vi "PicoScope4000aExampleBlock_PicoConnect.vi"() -> ()   [LabVIEW 2010]
doc: "This example demonstrates how to use the PicoScope Labview library to collect data using block mode with PicoConnect probe infomation."
uses:
  shared/PicoBuffers.ctl
  PicoScope4000aLib/PicoScope4000aAnalogChannelSettings_PicoConnect.ctl
  shared/Buffer and Transfer Settings.ctl
  shared/Acquisition Settings.ctl
panel:
  in  "Range":u32(ring)=4000 items=["10mV"=0, "20mV"=1, "50mV"=2, "100mV"=3, "200mV"=4, "500mV"=5, "1V"=6, "2V"=7, "5V"=8, "10V"=9, "20V"=10, "50V"=11, "100V"=12, "200V"=13, "1KV_2_5V"=6003, "1KV_5V"=6004, "1KV_12_5V"=6005, "1KV_25V"=6006, "1KV_50V"=6007, "1KV_125V"=6008, "1KV_250V"=6009, "1KV_500V"=6010, "1KV_1000V"=6011, "CURRENT_CLAMP_200A_2kA_1A"=4000, "CURRENT_CLAMP_200A_2kA_2A"=4001, "CURRENT_CLAMP_200A_2kA_5A"=4002, "CURRENT_CLAMP_200A_2kA_10A"=4003, "CURRENT_CLAMP_200A_2kA_20A"=4004, "CURRENT_CLAMP_200A_2kA_50A"=4005, "CURRENT_CLAMP_200A_2kA_100A"=4006, "CURRENT_CLAMP_200A_2kA_200A"=4007, "CURRENT_CLAMP_200A_2kA_500A"=4008, "CURRENT_CLAMP_200A_2kA_1000A"=4009, "CURRENT_CLAMP_200A_2kA_2000A"=4010, "CURRENT_CLAMP_40A_100mA"=5000, "CURRENT_CLAMP_40A_200mA"=5001, "CURRENT_CLAMP_40A_500mA"=5002, "CURRENT_CLAMP_40A_1A"=5003, "CURRENT_CLAMP_40A_2A"=5004, "CURRENT_CLAMP_40A_5A"=5005, "CURRENT_CLAMP_40A_10A"=5006, "CURRENT_CLAMP_40A_20A"=5007, "CURRENT_CLAMP_40A_40A"=5008, "CURRENT_CLAMP_2000ARMS_10A"=6500, "CURRENT_CLAMP_2000ARMS_20A"=6501, "CURRENT_CLAMP_2000ARMS_50A"=6502, "CURRENT_CLAMP_2000ARMS_100A"=6503, "CURRENT_CLAMP_2000ARMS_200A"=6504, "CURRENT_CLAMP_2000ARMS_500A"=6505, "CURRENT_CLAMP_2000ARMS_1000A"=6506, "CURRENT_CLAMP_2000ARMS_2000A"=6507, "CURRENT_CLAMP_2000ARMS_5000A"=6508, "x10_Probe_100mV"=32, "x10_Probe_200mV"=33, "x10_Probe_500mV"=34, "x10_Probe_1V"=35, "x10_Probe_2V"=36, "x10_Probe_5V"=37, "x10_Probe_10V"=38, "x10_Probe_20V"=39, "x10_Probe_50V"=40, "x10_Probe_100V"=41, "x10_Probe_200V"=42, "x10_Probe_500V"=43, "CURRENT_CLAMP_60A_2A"=10500, "CURRENT_CLAMP_60A_5A"=10501, "CURRENT_CLAMP_60A_10A"=10502, "CURRENT_CLAMP_60A_20A"=10503, "CURRENT_CLAMP_60A_50A"=10504, "CURRENT_CLAMP_60A_60A"=10505, "CURRENT_CLAMP_60A_V2_0_5A"=10600, "CURRENT_CLAMP_60A_V2_1A"=10601, "CURRENT_CLAMP_60A_V2_2A"=10602, "CURRENT_CLAMP_60A_V2_5A"=10603, "CURRENT_CLAMP_60A_V2_10A"=10604, "CURRENT_CLAMP_60A_V2_20A"=10605, "CURRENT_CLAMP_60A_V2_50A"=10606, "CURRENT_CLAMP_60A_V2_60A"=10607, "RESISTANCE_LEAD_NEG5_TO_20OHM"=7000, "RESISTANCE_LEAD_NEG50_TO_200OHM"=7001, "RESISTANCE_LEAD_NEG500_TO_2KOHM"=7002, "RESISTANCE_LEAD_NEG5K_TO_20KOHM"=7003, "RESISTANCE_LEAD_NEG50K_TO_LEAD_200KOHM"=7004, "RESISTANCE_LEAD_NEG500K_TO_LEAD_2MOHM"=7005, "RESISTANCE_LEAD_DIODE_TEST"=7006, "HT_NEG3_TO_5KV"=8950, "HT_NEG3_TO_10KV"=8951, "HT_NEG5_TO_20KV"=8952, "HT_NEG5_TO_50KV"=8953, "HT_NEG5_TO_100KV"=8954, "HT_NEG3_TO_5KV_INVERTED"=8955, "HT_NEG3_TO_10KV_INVERTED"=8956, "HT_NEG5_TO_20KV_INVERTED"=8957, "HT_NEG5_TO_50KV_INVERTED"=8958, "HT_NEG5_TO_100KV_INVERTED"=8959, "TEMPERATURE_NEG50_TO_150DEGC"=9000, "PRESSURE_SENSOR_-100k-150k_PASCALS"=9100, "PRESSURE_SENSOR_-100k_TO_400k_PASCALS"=9101, "PRESSURE_SENSOR_-200k_TO_800k_PASCALS"=9102, "PRESSURE_SENSOR_-400k_TO_1600k_PASCALS"=9103, "PRESSURE_SENSOR_-400k_TO_3400k_PASCALS"=9104, "PRESSURE_SENSOR_-150k_TO_1350k_PASCALS"=9105]
  in  "Trigger Settings":T1={"Trigger Enabled"=FALSE, "Trigger Source"=enum."Channel A", "Trigger Threshold (Volts/Probe units)"=0.0, "Trigger Direction"=2, "Trigger Delay (samples)"=0, "Auto Trigger Time (ms)"=1000} {"Trigger Direction" items=["Above", "Below", "Rising", "Falling", "Rising or Falling"]}
  out "Unit Info":T2
  out "minimumValue":sgl
  out "maximumValue":sgl
  out "Channel B":cluster{i32, dbl, "Data":dbl[]}[](graph)
  in  "Acquisition Settings":T3={"preTriggerSamples"=0, "postTriggerSamples"=5000000, "timebase"=5} {"postTriggerSamples" format="%_6p"; "preTriggerSamples" format="%_6p"}
  in  "Buffer and Transfer Settings":T4={"startIndex"=0, "Samples"=5000000, "Down Sample Ratio"=1, "Down-Sample Mode"=0} {"Down-Sample Mode" items=["RAW none"=2147483648, "None"=0, "Aggregate"=1, "Decimate"=2, "Average"=4]; "Down Sample Ratio" step=1; "Samples" format="%_6p"}
  out "Properties Panel":T5 {"Max Total Capture Time Available (sec)" format="%.3p"; "Sample Frequency" format="%.6p"; "Sample Rate" format="%.3p"; "Max Samples Available" format="%_6p"; "Total Capture Time (sec)" format="%.3p"}
  out "overflow":i16 format="%04b"
  out "Channel A":cluster{i32, dbl, "Data":dbl[]}(graph)
  in  "stop":bool
  out "ChB Probe":i32(ring) items=["CONNECT_PROBE_NONE"=0, "PROBE_D9_BNC"=4000, "PROBE_D9_2X_BNC"=4001, "PROBE_DIFFERENTIAL"=4002, "PROBE_CURRENT_CLAMP_200_2KA"=4003, "CONNECT_PROBE_CURRENT_CLAMP_40A"=4004, "CONNECT_PROBE_CAT3_HV_1KV"=4005, "CONNECT_PROBE_CURRENT_CLAMP_2000ARMS"=4006, "CONNECT_PROBE_INTELLIGENT"=-3, "CONNECT_PROBE_FAULT_PROBE"=-1, "CONNECT_PROBE_UNKNOWN_PROBE"=-2]
  in  "Channel A Settings":T6={"Enabled"=TRUE, "Coupling"=1, "Range"=0, "Analogue Offset"=0.0, "Bandwidth Limit"=0} {"Range" items=["10mV"=0, "20mV"=1, "50mV"=2, "100mV"=3, "200mV"=4, "500mV"=5, "1V"=6, "2V"=7, "5V"=8, "10V"=9, "20V"=10, "50V"=11, "100V"=12, "200V"=13, "1KV_2_5V"=6003, "1KV_5V"=6004, "1KV_12_5V"=6005, "1KV_25V"=6006, "1KV_50V"=6007, "1KV_125V"=6008, "1KV_250V"=6009, "1KV_500V"=6010, "1KV_1000V"=6011, "CURRENT_CLAMP_200A_2kA_1A"=4000, "CURRENT_CLAMP_200A_2kA_2A"=4001, "CURRENT_CLAMP_200A_2kA_5A"=4002, "CURRENT_CLAMP_200A_2kA_10A"=4003, "CURRENT_CLAMP_200A_2kA_20A"=4004, "CURRENT_CLAMP_200A_2kA_50A"=4005, "CURRENT_CLAMP_200A_2kA_100A"=4006, "CURRENT_CLAMP_200A_2kA_200A"=4007, "CURRENT_CLAMP_200A_2kA_500A"=4008, "CURRENT_CLAMP_200A_2kA_1000A"=4009, "CURRENT_CLAMP_200A_2kA_2000A"=4010, "CURRENT_CLAMP_40A_100mA"=5000, "CURRENT_CLAMP_40A_200mA"=5001, "CURRENT_CLAMP_40A_500mA"=5002, "CURRENT_CLAMP_40A_1A"=5003, "CURRENT_CLAMP_40A_2A"=5004, "CURRENT_CLAMP_40A_5A"=5005, "CURRENT_CLAMP_40A_10A"=5006, "CURRENT_CLAMP_40A_20A"=5007, "CURRENT_CLAMP_40A_40A"=5008, "CURRENT_CLAMP_2000ARMS_10A"=6500, "CURRENT_CLAMP_2000ARMS_20A"=6501, "CURRENT_CLAMP_2000ARMS_50A"=6502, "CURRENT_CLAMP_2000ARMS_100A"=6503, "CURRENT_CLAMP_2000ARMS_200A"=6504, "CURRENT_CLAMP_2000ARMS_500A"=6505, "CURRENT_CLAMP_2000ARMS_1000A"=6506, "CURRENT_CLAMP_2000ARMS_2000A"=6507, "CURRENT_CLAMP_2000ARMS_5000A"=6508, "x10_Probe_100mV"=32, "x10_Probe_200mV"=33, "x10_Probe_500mV"=34, "x10_Probe_1V"=35, "x10_Probe_2V"=36, "x10_Probe_5V"=37, "x10_Probe_10V"=38, "x10_Probe_20V"=39, "x10_Probe_50V"=40, "x10_Probe_100V"=41, "x10_Probe_200V"=42, "x10_Probe_500V"=43, "CURRENT_CLAMP_60A_2A"=10500, "CURRENT_CLAMP_60A_5A"=10501, "CURRENT_CLAMP_60A_10A"=10502, "CURRENT_CLAMP_60A_20A"=10503, "CURRENT_CLAMP_60A_50A"=10504, "CURRENT_CLAMP_60A_60A"=10505, "CURRENT_CLAMP_60A_V2_0_5A"=10600, "CURRENT_CLAMP_60A_V2_1A"=10601, "CURRENT_CLAMP_60A_V2_2A"=10602, "CURRENT_CLAMP_60A_V2_5A"=10603, "CURRENT_CLAMP_60A_V2_10A"=10604, "CURRENT_CLAMP_60A_V2_20A"=10605, "CURRENT_CLAMP_60A_V2_50A"=10606, "CURRENT_CLAMP_60A_V2_60A"=10607, "RESISTANCE_LEAD_NEG5_TO_20OHM"=7000, "RESISTANCE_LEAD_NEG50_TO_200OHM"=7001, "RESISTANCE_LEAD_NEG500_TO_2KOHM"=7002, "RESISTANCE_LEAD_NEG5K_TO_20KOHM"=7003, "RESISTANCE_LEAD_NEG50K_TO_LEAD_200KOHM"=7004, "RESISTANCE_LEAD_NEG500K_TO_LEAD_2MOHM"=7005, "RESISTANCE_LEAD_DIODE_TEST"=7006, "HT_NEG3_TO_5KV"=8950, "HT_NEG3_TO_10KV"=8951, "HT_NEG5_TO_20KV"=8952, "HT_NEG5_TO_50KV"=8953, "HT_NEG5_TO_100KV"=8954, "HT_NEG3_TO_5KV_INVERTED"=8955, "HT_NEG3_TO_10KV_INVERTED"=8956, "HT_NEG5_TO_20KV_INVERTED"=8957, "HT_NEG5_TO_50KV_INVERTED"=8958, "HT_NEG5_TO_100KV_INVERTED"=8959, "TEMPERATURE_NEG50_TO_150DEGC"=9000, "PRESSURE_SENSOR_-100k-150k_PASCALS"=9100, "PRESSURE_SENSOR_-100k_TO_400k_PASCALS"=9101, "PRESSURE_SENSOR_-200k_TO_800k_PASCALS"=9102, "PRESSURE_SENSOR_-400k_TO_1600k_PASCALS"=9103, "PRESSURE_SENSOR_-400k_TO_3400k_PASCALS"=9104, "PRESSURE_SENSOR_-150k_TO_1350k_PASCALS"=9105, "PICO_CONNECT_PROBE_OFF"=1024]; "Bandwidth Limit" items=["Full", "20kHz", "100kHz", "1MHz"]; "Coupling" items=["AC", "DC"]}
  in  "Channel B Settings":T6={"Enabled"=FALSE, "Coupling"=1, "Range"=0, "Analogue Offset"=0.0, "Bandwidth Limit"=0} {"Range" items=["10mV"=0, "20mV"=1, "50mV"=2, "100mV"=3, "200mV"=4, "500mV"=5, "1V"=6, "2V"=7, "5V"=8, "10V"=9, "20V"=10, "50V"=11, "100V"=12, "200V"=13, "1KV_2_5V"=6003, "1KV_5V"=6004, "1KV_12_5V"=6005, "1KV_25V"=6006, "1KV_50V"=6007, "1KV_125V"=6008, "1KV_250V"=6009, "1KV_500V"=6010, "1KV_1000V"=6011, "CURRENT_CLAMP_200A_2kA_1A"=4000, "CURRENT_CLAMP_200A_2kA_2A"=4001, "CURRENT_CLAMP_200A_2kA_5A"=4002, "CURRENT_CLAMP_200A_2kA_10A"=4003, "CURRENT_CLAMP_200A_2kA_20A"=4004, "CURRENT_CLAMP_200A_2kA_50A"=4005, "CURRENT_CLAMP_200A_2kA_100A"=4006, "CURRENT_CLAMP_200A_2kA_200A"=4007, "CURRENT_CLAMP_200A_2kA_500A"=4008, "CURRENT_CLAMP_200A_2kA_1000A"=4009, "CURRENT_CLAMP_200A_2kA_2000A"=4010, "CURRENT_CLAMP_40A_100mA"=5000, "CURRENT_CLAMP_40A_200mA"=5001, "CURRENT_CLAMP_40A_500mA"=5002, "CURRENT_CLAMP_40A_1A"=5003, "CURRENT_CLAMP_40A_2A"=5004, "CURRENT_CLAMP_40A_5A"=5005, "CURRENT_CLAMP_40A_10A"=5006, "CURRENT_CLAMP_40A_20A"=5007, "CURRENT_CLAMP_40A_40A"=5008, "CURRENT_CLAMP_2000ARMS_10A"=6500, "CURRENT_CLAMP_2000ARMS_20A"=6501, "CURRENT_CLAMP_2000ARMS_50A"=6502, "CURRENT_CLAMP_2000ARMS_100A"=6503, "CURRENT_CLAMP_2000ARMS_200A"=6504, "CURRENT_CLAMP_2000ARMS_500A"=6505, "CURRENT_CLAMP_2000ARMS_1000A"=6506, "CURRENT_CLAMP_2000ARMS_2000A"=6507, "CURRENT_CLAMP_2000ARMS_5000A"=6508, "x10_Probe_100mV"=32, "x10_Probe_200mV"=33, "x10_Probe_500mV"=34, "x10_Probe_1V"=35, "x10_Probe_2V"=36, "x10_Probe_5V"=37, "x10_Probe_10V"=38, "x10_Probe_20V"=39, "x10_Probe_50V"=40, "x10_Probe_100V"=41, "x10_Probe_200V"=42, "x10_Probe_500V"=43, "CURRENT_CLAMP_60A_2A"=10500, "CURRENT_CLAMP_60A_5A"=10501, "CURRENT_CLAMP_60A_10A"=10502, "CURRENT_CLAMP_60A_20A"=10503, "CURRENT_CLAMP_60A_50A"=10504, "CURRENT_CLAMP_60A_60A"=10505, "CURRENT_CLAMP_60A_V2_0_5A"=10600, "CURRENT_CLAMP_60A_V2_1A"=10601, "CURRENT_CLAMP_60A_V2_2A"=10602, "CURRENT_CLAMP_60A_V2_5A"=10603, "CURRENT_CLAMP_60A_V2_10A"=10604, "CURRENT_CLAMP_60A_V2_20A"=10605, "CURRENT_CLAMP_60A_V2_50A"=10606, "CURRENT_CLAMP_60A_V2_60A"=10607, "RESISTANCE_LEAD_NEG5_TO_20OHM"=7000, "RESISTANCE_LEAD_NEG50_TO_200OHM"=7001, "RESISTANCE_LEAD_NEG500_TO_2KOHM"=7002, "RESISTANCE_LEAD_NEG5K_TO_20KOHM"=7003, "RESISTANCE_LEAD_NEG50K_TO_LEAD_200KOHM"=7004, "RESISTANCE_LEAD_NEG500K_TO_LEAD_2MOHM"=7005, "RESISTANCE_LEAD_DIODE_TEST"=7006, "HT_NEG3_TO_5KV"=8950, "HT_NEG3_TO_10KV"=8951, "HT_NEG5_TO_20KV"=8952, "HT_NEG5_TO_50KV"=8953, "HT_NEG5_TO_100KV"=8954, "HT_NEG3_TO_5KV_INVERTED"=8955, "HT_NEG3_TO_10KV_INVERTED"=8956, "HT_NEG5_TO_20KV_INVERTED"=8957, "HT_NEG5_TO_50KV_INVERTED"=8958, "HT_NEG5_TO_100KV_INVERTED"=8959, "TEMPERATURE_NEG50_TO_150DEGC"=9000, "PRESSURE_SENSOR_-100k-150k_PASCALS"=9100, "PRESSURE_SENSOR_-100k_TO_400k_PASCALS"=9101, "PRESSURE_SENSOR_-200k_TO_800k_PASCALS"=9102, "PRESSURE_SENSOR_-400k_TO_1600k_PASCALS"=9103, "PRESSURE_SENSOR_-400k_TO_3400k_PASCALS"=9104, "PRESSURE_SENSOR_-150k_TO_1350k_PASCALS"=9105, "PICO_CONNECT_PROBE_OFF"=1024]; "Bandwidth Limit" items=["Full", "20kHz", "100kHz", "1MHz"]; "Coupling" items=["AC", "DC"]}
  out "ChA Probe":i32(ring) items=["CONNECT_PROBE_NONE"=0, "PROBE_D9_BNC"=4000, "PROBE_D9_2X_BNC"=4001, "PROBE_DIFFERENTIAL"=4002, "PROBE_CURRENT_CLAMP_200_2KA"=4003, "CONNECT_PROBE_CURRENT_CLAMP_40A"=4004, "CONNECT_PROBE_CAT3_HV_1KV"=4005, "CONNECT_PROBE_CURRENT_CLAMP_2000ARMS"=4006, "CONNECT_PROBE_INTELLIGENT"=-3, "CONNECT_PROBE_FAULT_PROBE"=-1, "CONNECT_PROBE_UNKNOWN_PROBE"=-2]
  out "USB 3.0 on non-USB 3.0 port":bool=TRUE
  out "USB powered":bool=TRUE
  in  "Resolution":u32(ring)=1 items=["12-bit"=1, "14-bit"=2]
  in  "Serial Number":string
  in  "Open using Serial Number":bool
  # "Note: Probe Channel scaling is done in ADCtoVolts.vi"
  # "ps4000aGetAnalogueOffset"
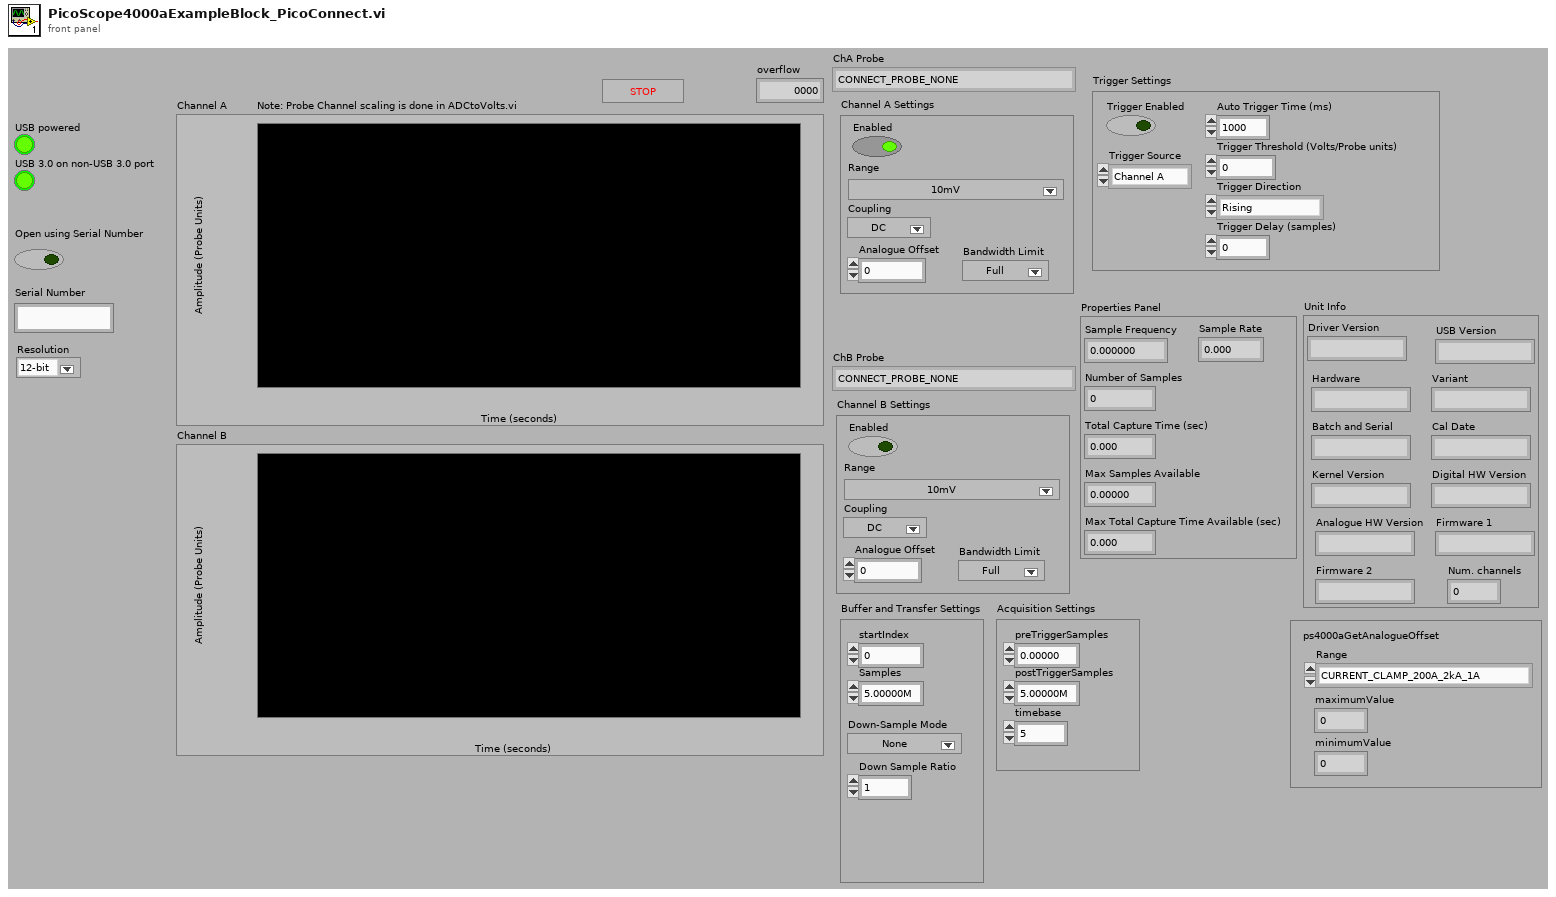
[diagram p1: front panel]
types:
  T1 = cluster{"Trigger Enabled":bool, "Trigger Source":enum16{"Channel A", "Channel B", "Channel C", "Channel D", "Channel E", "Channel F", "Channel G", "Channel H"}, "Trigger Threshold (Volts/Probe units)":dbl, "Trigger Direction":u16, "Trigger Delay (samples)":u32, "Auto Trigger Time (ms)":i16}
  T2 = cluster{"Driver Version":string, "USB Version":string, "Hardware":string, "Variant":string, "Batch and Serial":string, "Cal Date":string, "Kernel Version":string, "Digital HW Version":string, "Analogue HW Version":string, "Firmware 1":string, "Firmware 2":string, "Num. channels":i16}
  T3 = typedef "Acquisition Settings.ctl" = cluster{"preTriggerSamples":u64, "postTriggerSamples":u64, "timebase":u32}
  T4 = typedef "Buffer and Transfer Settings.ctl" = cluster{"startIndex":u64, "Samples":u64, "Down Sample Ratio":u64, "Down-Sample Mode":u32}
  T5 = cluster{"Sample Frequency":dbl, "Sample Rate":dbl, "Max Samples Available":u64, "Number of Samples":u64, "Total Capture Time (sec) ":dbl, "Max Total Capture Time Available (sec)":dbl}
  T6 = typedef "PicoScope4000aAnalogChannelSettings_PicoConnect.ctl" = cluster{"Enabled":bool, "Coupling":i16, "Range":u32, "Analogue Offset":sgl, "Bandwidth Limit":u32}
  T7 = typedef "PicoBuffers.ctl" = cluster{"Max Buffer Pointers":u64[][][], "Min Buffer Pointers":u64[][][], "StreamingDataInfo":cluster{"Channel":u32, "Down-Sample Mode":u32, "PICO_DATA_TYPE":enum32{"PICO_INT8_T", "PICO_INT16_T", "PICO_INT32_T", "PICO_UINT32_T", "PICO_INT64_T", ""}, "Samples":i32, "bufferIndex":u64, "startIndex":i32, "overflow":i16}[][]}
  T8 = cluster{"probeNumber":i32, bool, "channel":i32, "enabled":i16, "probeName":i32, "requiresPower":i8, "isPowered":i8, "probeOff":i32, "rangeFirst":i32, "rangeLast":i32, "rangeCurrent":i32, "couplingFirst":i32, "couplingLast":i32, "couplingCurrent":i32, "filterFlags":i32, "filterCurrent":i32, "defaultFilter":i32}[]
  T9 = typedef "PicoScope4000aAnalogChannelSettings.ctl" = cluster{"Enabled":bool, "Coupling":i16, "Range":u32, "Analogue Offset":sgl, "Bandwidth Limit":u32}
  T10 = cluster{"Probe Info":cluster{"Ch Min Limit":dbl, "Ch Max Limit":dbl, "Probe Name":i32}, "Channel A Settings ":T9}
  T11 = cluster{"Channel A Buffer":i16[], "Channel B Buffer":i16[], "Channel C Buffer":i16[], "Channel D Buffer":i16[], "Channel E Buffer":i16[], "Channel F Buffer":i16[], "Channel G Buffer":i16[], "Channel H Buffer":i16[], "Port 0 Buffer":i16[], "Port 1 Buffer":i16[]}[]
  T12 = cluster{"Channel A Buffer":i16[], "Channel B Buffer":i16[], "Channel C Buffer":i16[], "Channel D Buffer":i16[], "Channel E Buffer":i16[], "Channel F Buffer":i16[], "Channel G Buffer":i16[], "Channel H Buffer":i16[], "Port 0 Buffer":i16[], "Port 1 Buffer":i16[]}
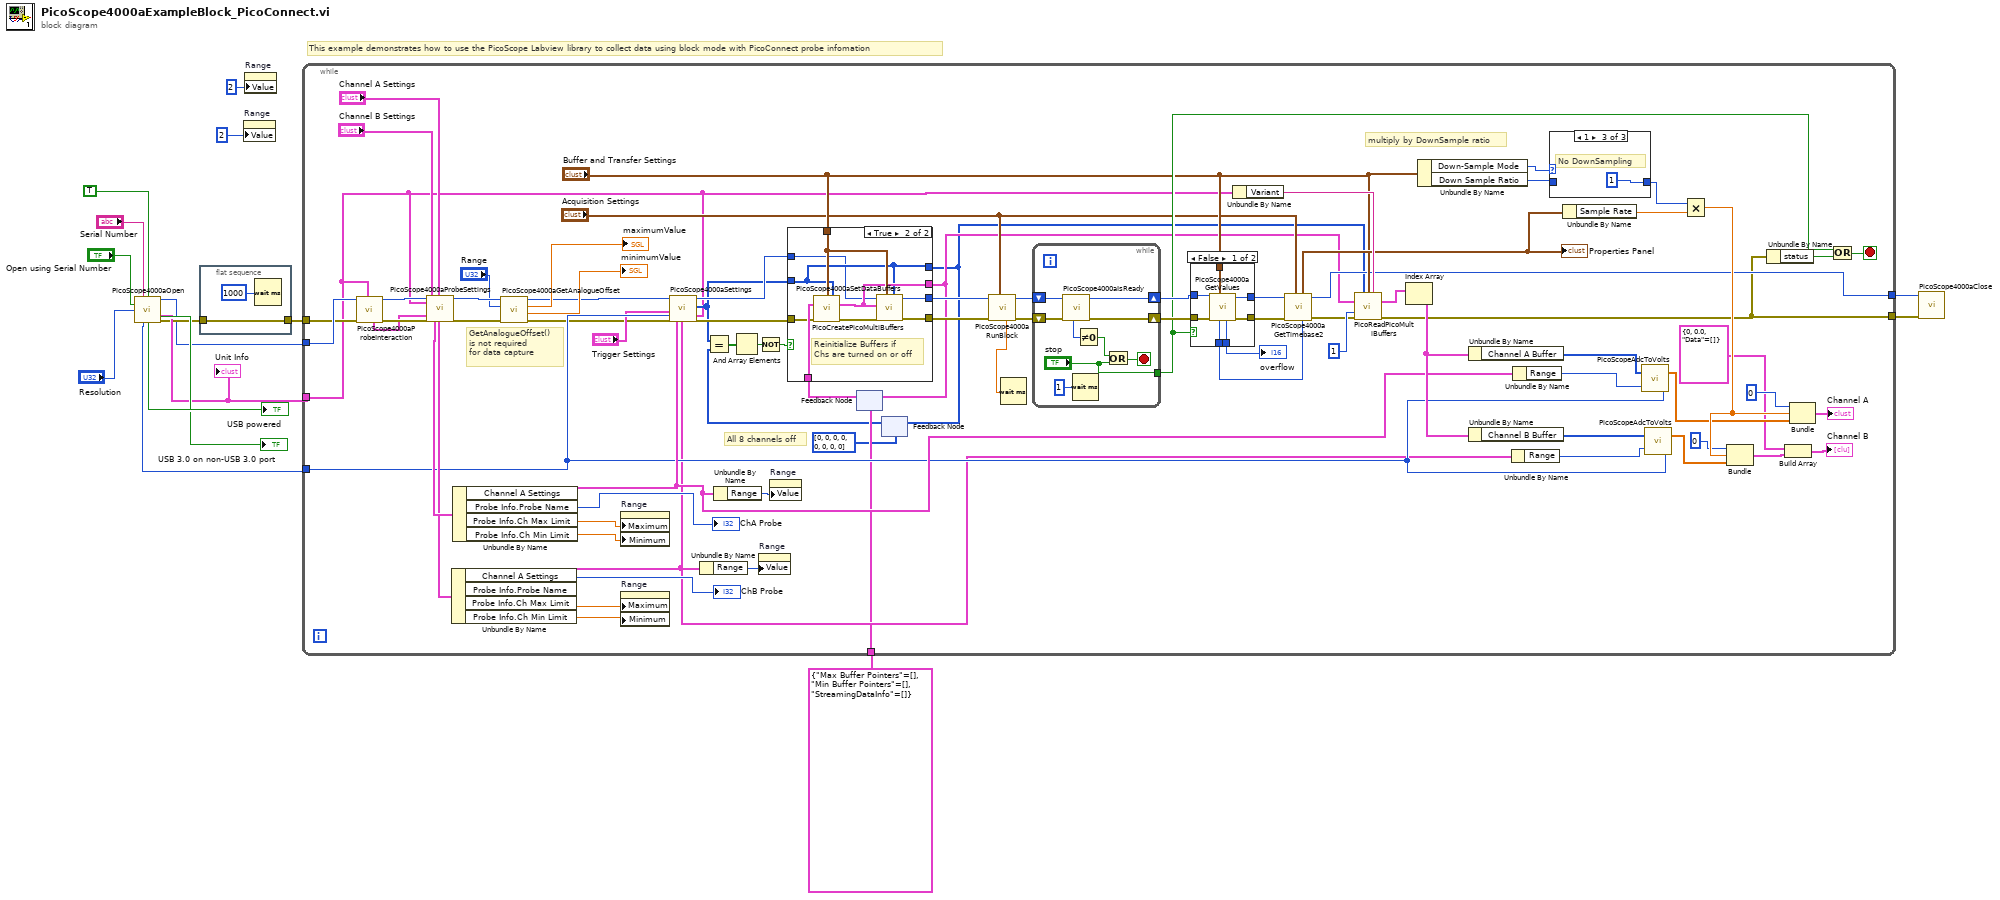
[diagram p0: block diagram]
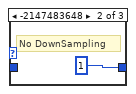
[diagram p5: hidden frame]
diagram:
  # "This example demonstrates how to use the PicoScope Labview library to collect data using block mode with PicoConnect probe infomation"
  n1 = call "PicoScope4000aOpen.vi"("Serial Number"="Serial Number", "setProbeInteractionCallback"=TRUE, "Use Serial Number"="Open using Serial Number", "Resolution"="Resolution") -> ("handle"=w1:i16, "Unit Info"=w11:T2, "Max ADC value"=w12:i16, "USB powered"=→"USB powered":bool, "USB 3.0 on non-USB 3.0 port"=→"USB 3.0 on non-USB 3.0 port":bool, "error out"=w2:errorcluster)  [unwired: 4 in, 2 out]
  "Unit Info" <- w11
  n2 = flat-sequence {
    tunnel: [w17] -> w4
    tunnel: w2 -> [w17]
    frame #0 {
      n3 = Wait (ms)(milliseconds to wait=u32 1000) -> ()  [unwired: 1 out]
    }
  }
  n4 = property on="Range" class="Ring (strict)"("Value"=u32 2) -> ()  [unwired: 2 in, 2 out]
  n5 = property on="Range" class="Ring (strict)"("Value"=u32 2) -> ()  [unwired: 2 in, 2 out]
  n6 = while {
    tunnel: w1 -> [w100]
    tunnel: w4 -> [w99]
    tunnel: w11 -> [w19]
    tunnel: w12 -> [w51]
    tunnel: [w55] -> w8
    tunnel: T7 {"Max Buffer Pointers"=[], "Min Buffer Pointers"=[], "StreamingDataInfo"=[]} ("Data Pointers") -> [w48]
    tunnel: [w27] -> w3
    stop <- w56 stop-if-true
    # "GetAnalogueOffset()\nis not required\nfor data capture"
    # "All 8 channels off"
    # "multiply by DownSample ratio"
    n7 = call "PicoScope4000aProbeInteraction.vi"("Device Info"=w19, "error in"=w99, "handle in"=w100) -> ("error out"=w97:errorcluster, "handle out"=w98:i16, "Output Probe Array"=w96:T8)  [unwired: 5 in, 1 out]
    n8 = call "PicoScope4000aProbeSettings.vi"("handle in"=w98, "Device Info"=w19, "Probe Input Array"=w96, "error in (no error)"=w97, "Channel A Settings"="Channel A Settings", "Channel B Settings"="Channel B Settings") -> ("ChA"=w95:T10, "ChB"=w94:T10, "handle out"=w36:i16, "error out"=w35:errorcluster)  [unwired: 8 in, 2 out]
    n9 = Unbundle By Name(w94) -> ("Channel A Settings"=w49:T9, "Probe Info.Probe Name"=→"ChB Probe":i32, "Probe Info.Ch Max Limit"=w28:dbl, "Probe Info.Ch Min Limit"=w29:dbl)
    n10 = Unbundle By Name(w95) -> ("Channel A Settings"=w52:T9, "Probe Info.Probe Name"=→"ChA Probe":i32, "Probe Info.Ch Max Limit"=w31:dbl, "Probe Info.Ch Min Limit"=w30:dbl)
    n11 = call "PicoScope4000aGetAnalogueOffset.vi"("error in (no error)"=w35, "Range"="Range", "handle in"=w36) -> ("error out"=w24:errorcluster, "minimumValue"=→"minimumValue":sgl, "maximumValue"=→"maximumValue":sgl, "handle out"=w23:i16)  [unwired: 5 in]
    n12 = property on="Range" class="Ring (strict)"("Maximum"=w31, "Minimum"=w30) -> ()  [unwired: 2 in, 2 out]
    n13 = property on="Range" class="Ring (strict)"("Maximum"=w28, "Minimum"=w29) -> ()  [unwired: 2 in, 2 out]
    n14 = call "PicoScope4000aSettings.vi"("handle in"=w23, "Trigger Settings"="Trigger Settings", "Max ADC value"=w51, "error in"=w24, "Channel A Settings"=w52, "Channel B Settings"=w49, "Unit Info"=w19) -> ("handle out"=w21:i16, "Enabled array"=w20:i16[], "error out"=w22:errorcluster)  [unwired: 10 in]
    n15 = Unbundle By Name(w49) -> ("Range"=w89:u32)
    n16 = Unbundle By Name(w52) -> ("Range"=w90:u32)
    n17 = property on="Range" class="Ring (strict)"("Value"=w89) -> ()  [unwired: 2 in, 2 out]
    n18 = property on="Range" class="Ring (strict)"("Value"=w90) -> ()  [unwired: 2 in, 2 out]
    n19 = feedback #1(w48) -> (w54:T7)
    n20 = feedback #2(i16[] [0, 0, 0, 0, 0, 0, 0, 0] ("Enabled array")) -> (w45:i16[])
    n21 = Equal?(x=w20, y=w45) -> (x = y?=w46:bool[])
    n22 = And Array Elements(Boolean array=w46) -> (logical AND=w42:bool)
    n23 = Not(x=w42) -> (.not. x?=w43:bool)
    n24 = case shown="True" w43 {
      tunnel: [w103 w112] -> w60
      tunnel: [w101 w111] -> w59
      tunnel: "Buffer and Transfer Settings" -> [_ w110]
      tunnel: [w102 w106] -> w47
      tunnel: [w104 w109] -> w53
      tunnel: w54 -> [w104 w108]
      tunnel: w22 -> [w103 w107]
      tunnel: w20 -> [w102 w106]
      tunnel: w21 -> [w101 w105]
      frame False {
      }
      frame True {
        # "Reinitialize Buffers if\nChs are turned on or off"
        n25 = call "PicoCreatePicoMultiBuffers.vi"("Buffer and Transfer Settings"=w110, "enabled array"=w106, "Data Pointers In"=w108, "error in (no error)"=w107) -> ("Data Pointers"=w109:T7, "error out"=w113:errorcluster)  [unwired: 10 in]
        n26 = call "PicoScope4000aSetDataBuffers.vi"("enabled array"=w106, "Buffer and Transfer Settings"=w110, "error in (no error)"=w113, "Data Pointers In"=w109, "handle in"=w105) -> ("error out"=w112:errorcluster, "handle out"=w111:i16)  [unwired: 5 in]
      }
    }
    n27 = feedback-in #1(w53) -> ()
    n28 = feedback-in #2(w47) -> ()
    n29 = call "PicoScope4000aRunBlock.vi"("Acquisition Settings"="Acquisition Settings", "error in (no error)"=w60, "handle in"=w59) -> ("error out"=w82:errorcluster, "handle out"=w81:i16, "timeIndisposedMs"=w32:dbl)  [unwired: 5 in, 1 out]
    n30 = Wait (ms)(milliseconds to wait=w32) -> ()  [unwired: 1 out]
    n31 = while {
      shift-right: [w130] -> w68
      shift-left: w82 -> [w131]
      shift-right: [w129] -> w69
      shift-left: w81 -> [w128]
      tunnel: ["stop"] -> w67
      stop <- w125 stop-if-true
      n32 = call "PicoScope4000aIsReady.vi"("error in (no error)"=w131, "handle in"=w128) -> ("error out"=w130:errorcluster, "handle out"=w129:i16, "ready"=w127:i16)  [unwired: 7 in]
      n33 = Wait (ms)(milliseconds to wait=u32 1) -> ()  [unwired: 1 out]
      n34 = Not Equal To 0?(x=w127) -> (x != 0?=w126:bool)
      n35 = Or(x=w126, y="stop") -> (x .or. y?=w125:bool)
    }
    n36 = case shown="False" w67 {
      tunnel: w68 -> [w120 w121]
      tunnel: w69 -> [w119 w122]
      tunnel: [w118 w122] -> w61
      tunnel: [w117 w121] -> w62
      tunnel: "Buffer and Transfer Settings" -> [w116 _]
      tunnel: [w115 _] -> w66
      tunnel: [w114 _] -> w65
      frame False {
        n37 = call "PicoScope4000aGetValues.vi"("Buffer and Transfer Settings"=w116, "error in (no error)"=w120, "handle in"=w119) -> ("error out"=w117:errorcluster, "handle out"=w118:i16, "overflow"=w115:i16, "noOfSamples"=w114:u64)  [unwired: 5 in]
      }
      frame True {
      }
    }
    "overflow" <- w66
    n38 = Unbundle By Name(w19) -> ("Variant"=w79:string)
    n39 = call "PicoScope4000aGetTimebase2.vi"("Number of Samples"=w65, "Acquisition Settings"="Acquisition Settings", "error in (no error)"=w62, "handle in"=w61) -> ("error out"=w63:errorcluster, "handle out"=w55:i16, "Properties Panel"=w64:T5)  [unwired: 5 in]
    "Properties Panel" <- w64
    n40 = call "PicoReadPicoMultiBuffers.vi"("enabled array"=w47, "Buffer and Transfer Settings"="Buffer and Transfer Settings", "Variant"=w79, "Data Pointers"=w53, "No of Buffers"=1, "error in (no error)"=w63) -> ("MultiBuffers (Max or non-aggregated)"=w87:T11, "error out"=w27:errorcluster)  [unwired: 7 in, 1 out]
    n41 = Index Array(array=w87) -> (element=w70:T12)  [unwired: 1 in]
    n42 = Unbundle By Name("Buffer and Transfer Settings") -> ("Down-Sample Mode"=w85:u32, "Down Sample Ratio"=w86:u64)
    n43 = Unbundle By Name(w70) -> ("Channel A Buffer"=w71:i16[])
    n44 = Unbundle By Name(w70) -> ("Channel B Buffer"=w74:i16[])
    n45 = Unbundle By Name(w49) -> ("Range"=w50:u32)
    n46 = Unbundle By Name(w52) -> ("Range"=w76:u32)
    n47 = case shown="1" w85 {
      tunnel: [w132 u64 1 ("Down Sample Ratio") u64 1 ("Down Sample Ratio")] -> w83
      tunnel: w86 -> [w132 _ _]
      frame Default {
      }
      frame -2147483648 {
        # "No DownSampling"
      }
      frame 1 {
        # "No DownSampling"
      }
    }
    n48 = Unbundle By Name(w64) -> ("Sample Rate"=w80:dbl)
    n49 = call "PicoScopeAdcToVolts.vi"("Max_adc"=w51, "Range Index"=w76, "Data"=w71) -> ("Data"=w72:dbl[])
    n50 = call "PicoScopeAdcToVolts.vi"("Max_adc"=w51, "Range Index"=w50, "Data"=w74) -> ("Data"=w73:dbl[])
    n51 = Multiply(x=w83, y=w80) -> (x*y=w84:dbl)
    n52 = Bundle(0, w84, "Data"=w73) -> (w38:cluster{i32, dbl, "Data":dbl[]})  [unwired: 1 in]
    n53 = Unbundle By Name(w27) -> ("status"=w41:bool)
    n54 = Build Array(cluster{i32, dbl, "Data":dbl[]} {0, 0.0, "Data"=[]} ("element"), w38) -> (→"Channel B":cluster{i32, dbl, "Data":dbl[]}[])
    n55 = Bundle(0, w84, "Data"=w72) -> (→"Channel A":cluster{i32, dbl, "Data":dbl[]})  [unwired: 1 in]
    n56 = Or(x=w67, y=w41) -> (x .or. y?=w56:bool)
  }
  n57 = call "PicoScope4000aClose.vi"("error in (no error)"=w3, "handle in"=w8) -> ()  [unwired: 7 in, 2 out]
